vi "take-sample.vi"(10 "notifier out":refnum<notifier>) -> ()   [LabVIEW 2012]
uses:
  <vilib>/GPower/VIRegister/Library/SubVIs/FindRegisterData.vi
  <vilib>/GPower/VIRegister/Library/SubVIs/ReadSub.vi
  <vilib>/GPower/VIRegister/Library/SubVIs/WriteSub.vi
  <vilib>/GPower/VIRegister/Library/QManager/GetRegisterData.vi
  <vilib>/GPower/Error/Library/SetError.vi
  <vilib>/GPower/Error/Library/FilterCodes.vi
  <vilib>/GPower/Error/Library/Filter/FilterMulti.vi
  <vilib>/GPower/VIRegister/Library/QManager/QManagerAction.vi
  <vilib>/GPower/Error/Library/ErrorType.vi
  <vilib>/GPower/Error/Library/SplitAppended.vi
  <vilib>/GPower/Error/Library/SubVIs/ExplanationToError.vi
  <vilib>/GPower/VIRegister/Library/QManager/GetQName.vi
  <vilib>/GPower/VIRegister/Library/QManager/StartQManager.vi
  <vilib>/Utility/error.llb/Trim Whitespace.vi
  <vilib>/dlg_ctls.llb/Space Constant.vi
  <vilib>/Utility/error.llb/Error Code Database.vi
  <vilib>/GPower/Error/Library/SubVIs/SetStatus.vi
  <vilib>/GPower/Error/Library/AppendErrors.vi
  <vilib>/GPower/Error/Library/Append/AppendSingle.vi
  <vilib>/GPower/VIRegister/VIRegister.lvlib
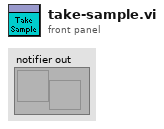
[diagram p1: front panel]
types:
  T1 = cluster{"data":string, "timestamp":cluster{"tv_sec":u32, "tv_usec":u32}}
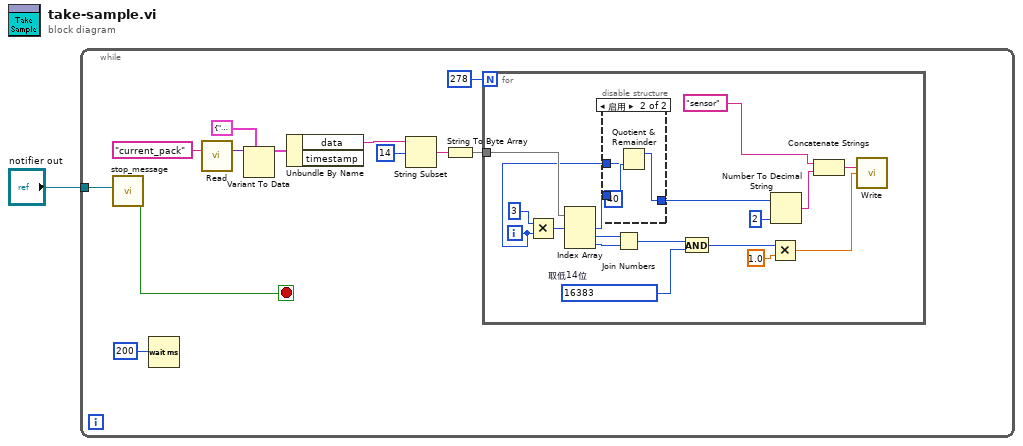
[diagram p0: block diagram]
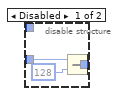
[diagram p2: hidden frame]
diagram:
  n1 = while {
    tunnel: "notifier out" -> [w9]
    stop <- w8 stop-if-true
    n2 = call "stop_message.vi"("notifier"=w9) -> ("Exit？"=w8:bool)  [unwired: 9 in, 1 out]
    n3 = Wait (ms)(milliseconds to wait=u32 200 ("等待时间（毫秒）")) -> ()  [unwired: 1 out]
    n4 = call <vilib>:"Read.vi"("Register name"="current_pack") -> ("Register value"=w12:variant)  [unwired: 11 in, 3 out]
    n5 = Variant To Data(type=T1 {"data"="", "timestamp"={"tv_sec"=0, "tv_usec"=0}} ("输出簇"), Variant=w12) -> (data=w10:T1)  [unwired: 1 in, 1 out]
    n6 = Unbundle By Name(w10) -> ("data"=w5:string)  [unwired: 1 out]
    n7 = String Subset(string=w5, offset (0)=14 ("偏移量(0)")) -> (substring=w3:string)  [unwired: 1 in]
    n8 = String To Byte Array(string=w3) -> (unsigned byte array=w6:u8[])
    n9 = for {
      N: 278 -> [_]
      tunnel: w6 -> [w30]
      i -> [w16]
      w22 = u16 16383  # 取低14位
      n10 = Multiply(x=3, y=w16) -> (x*y=w28:i32)
      n11 = Index Array(array=w30, index #1=w28) -> (element #1=w27:u8, element #2=w25:u8, element #3=w24:u8)  [unwired: 2 in]
      n12 = disable-structure shown="启用" {
        disable-tunnel: w27 -> [w33 _]
        disable-tunnel: [w31 w34] -> w18
        disable-tunnel: w16 -> [_ w35]
        frame Disabled {
          n13 = Subtract(x=w33, y=u8 128) -> (x-y=w31:u8)
        }
        frame Enabled {
          n14 = Quotient & Remainder(x=w35, y=40) -> (x-y*floor(x/y)=w34:i32)  [unwired: 1 out]
        }
      }
      n15 = Join Numbers(hi=w25, lo=w24) -> ((hi.lo)=w23:u16)
      n16 = And(x=w23, y=w22) -> (x .and. y?=w21:u16)
      n17 = Multiply(x=w21, y=sgl 1.0) -> (x*y=w19:sgl)
      n18 = Number To Decimal String(number=w18, width (-)=i16 2 ("宽度(-)")) -> (decimal integer string=w26:string)
      n19 = Concatenate Strings("sensor" ("Register name"), w26) -> (w17:string)
      n20 = call <vilib>:"Write.vi"("Register name"=w17, "Register value"=w19) -> ()  [unwired: 11 in, 3 out]
    }
  }
